vi "Convert Font To Font Object.vi"(8 "error in (no error)":errorcluster, 10 "Font":T1={"Name"="Calibri", "Size"=12, "Bold"=FALSE, "Italic"=FALSE, "Underline"=18, "Strike"=FALSE, "Color"=0} {"Underline" items=["Single"=1, "Words"=2, "Double"=3, "Thick"=4, "Dotted"=5, "DottedHeavy"=6, "Dash"=7, "DashedHeavy"=8, "DashLong"=9, "DashLongHeavy"=10, "DotDash"=11, "DashDotHeavy"=12, "DotDotDash"=13, "DashDotDotHeavy"=14, "Wave"=15, "WavyHeavy"=16, "WavyDouble"=17, "None"=18]}) -> (0 "error out":errorcluster, 3 "Font Object":refnum<class "Style.lvclass">)   [LabVIEW 2020, in "Styles.lvlib"]
uses:
  Styles.lvlib
  Style/Style.lvclass
  Title/Title.lvclass
  Heading 1/Heading 1.lvclass
  Heading 2/Heading 2.lvclass
  Heading 3/Heading 3.lvclass
  D:/Benjamin/Documents/Perso/Code/WC/LabVIEW_NPOI/src/Font/Font/Style.lvclass
  D:/Benjamin/Documents/Perso/Code/WC/LabVIEW_NPOI/src/Font/Title/Title.lvclass
  D:/Benjamin/Documents/Perso/Code/WC/LabVIEW_NPOI/src/Font/Heading/Heading.lvclass
  D:/Benjamin/Documents/Perso/Code/WC/LabVIEW_NPOI/src/Font/Heading 1/Heading 1.lvclass
  D:/Benjamin/Documents/Perso/Code/WC/LabVIEW_NPOI/src/Font/Heading 2/Heading 2.lvclass
  D:/Benjamin/Documents/Perso/Code/WC/LabVIEW_NPOI/src/Font/Heading 3/Heading 3.lvclass
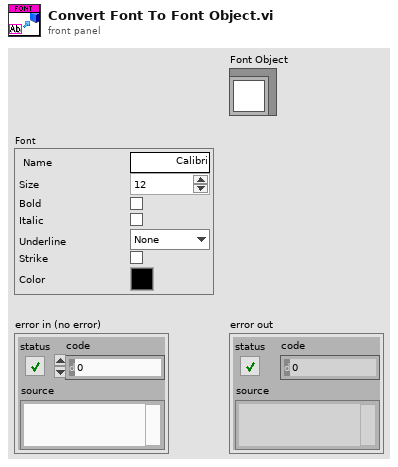
[diagram p1: front panel]
types:
  T1 = cluster{"Name":string, "Size":i32, "Bold":bool, "Italic":bool, "Underline":i32, "Strike":bool, "Color":u32}
  T2 = typedef "Styles.lvlib/Style.lvclass/Underline--ring.ctl" = i32
  T3 = cluster{"Public VIs:Properties:Name":string, "Public VIs:Properties:Size":i32, "Public VIs:Properties:Bold":bool, "Public VIs:Properties:Italic":bool, "Public VIs:Properties:Underline":T2, "Public VIs:Properties:Strike":bool, "Public VIs:Properties:Color":u32}
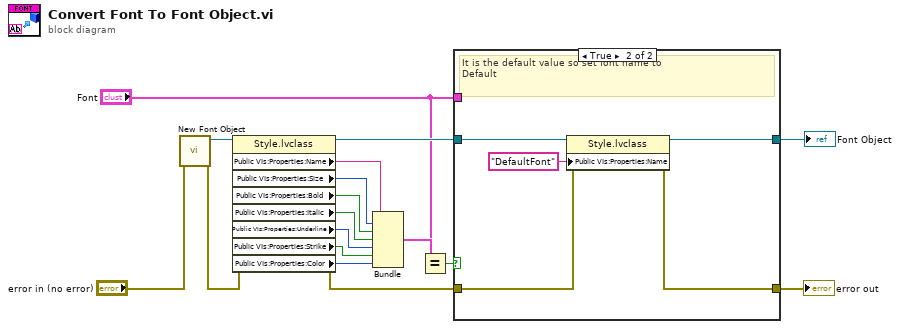
[diagram p0: block diagram]
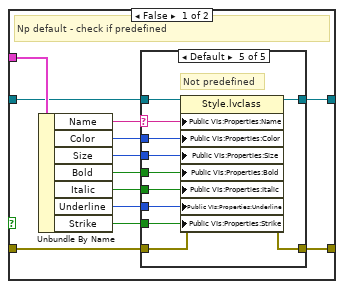
[diagram p2: hidden frame]
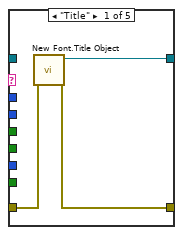
[diagram p3: hidden frame]
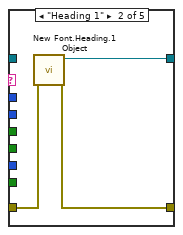
[diagram p4: hidden frame]
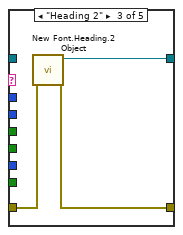
[diagram p5: hidden frame]
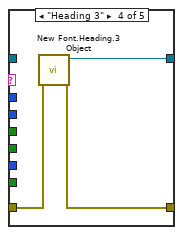
[diagram p6: hidden frame]
diagram:
  n1 = call "New Font Object.vi"("error in (no error)"="error in (no error)") -> ("error out"=w2:errorcluster, "Font out"=w4:refnum<class "Style.lvclass">)  [unwired: 9 in]
  n2 = property class="Style.lvclass"(reference=w4, error in=w2) -> (reference out=w14:refnum<class "Style.lvclass">, error out=w5:errorcluster, "Public VIs:Properties:Name"=w13:string, "Public VIs:Properties:Size"=w12:i32, "Public VIs:Properties:Bold"=w11:bool, "Public VIs:Properties:Italic"=w10:bool, "Public VIs:Properties:Underline"=w9:T2, "Public VIs:Properties:Strike"=w8:bool, "Public VIs:Properties:Color"=w7:u32)
  n3 = Bundle("Public VIs:Properties:Name"=w13, "Public VIs:Properties:Size"=w12, "Public VIs:Properties:Bold"=w11, "Public VIs:Properties:Italic"=w10, "Public VIs:Properties:Underline"=w9, "Public VIs:Properties:Strike"=w8, "Public VIs:Properties:Color"=w7) -> (w6:T3)  [unwired: 1 in]
  n4 = Equal?(x=w6, y="Font") -> (x = y?=w17:bool)
  n5 = case shown="True" w17 {
    tunnel: "Font" -> [w23 _]
    tunnel: [w22 w56] -> w16
    tunnel: w14 -> [w19 w57]
    tunnel: [w21 w54] -> w15
    tunnel: w5 -> [w18 w53]
    frame False {
      # "Np default - check if predefined"
      n6 = Unbundle By Name(w23) -> ("Name"=w20:string, "Color"=w28:u32, "Size"=w27:i32, "Bold"=w26:bool, "Italic"=w25:bool, "Underline"=w24:i32, "Strike"=w29:bool)
      n7 = case shown="Default" w20 {
        selector: w20 -> [_ _ _ _ w44]
        tunnel: w29 -> [_ _ _ _ w52]
        tunnel: w28 -> [_ _ _ _ w51]
        tunnel: w27 -> [_ _ _ _ w50]
        tunnel: w26 -> [_ _ _ _ w49]
        tunnel: w25 -> [_ _ _ _ w48]
        tunnel: w24 -> [_ _ _ _ w47]
        tunnel: [w32 w35 w38 w41 w46] -> w22
        tunnel: [w30 w33 w37 w39 w45] -> w21
        tunnel: w19 -> [_ _ _ _ w43]
        tunnel: w18 -> [w31 w34 w36 w40 w42]
        frame "Title" {
          n8 = call "New Font.Title Object.vi"("error in (no error)"=w31) -> ("error out"=w30:errorcluster, "Title out"=w32:refnum<class "Title.lvclass">)  [unwired: 9 in]
        }
        frame "Heading 1" {
          n9 = call "New Font.Heading.1 Object.vi"("error in (no error)"=w34) -> ("error out"=w33:errorcluster, "Heading 1 out"=w35:refnum<class "Heading 1.lvclass">)  [unwired: 9 in]
        }
        frame "Heading 2" {
          n10 = call "New Font.Heading.2 Object.vi"("error in (no error)"=w36) -> ("error out"=w37:errorcluster, "Heading 2 out"=w38:refnum<class "Heading 2.lvclass">)  [unwired: 9 in]
        }
        frame "Heading 3" {
          n11 = call "New Font.Heading.3 Object.vi"("error in (no error)"=w40) -> ("error out"=w39:errorcluster, "Heading 3 out"=w41:refnum<class "Heading 3.lvclass">)  [unwired: 9 in]
        }
        frame Default {
          # "Not predefined"
          # "Not predefined"
          n12 = property class="Style.lvclass"(reference=w43, error in=w42, "Public VIs:Properties:Name"=w44, "Public VIs:Properties:Color"=w51, "Public VIs:Properties:Size"=w50, "Public VIs:Properties:Bold"=w49, "Public VIs:Properties:Italic"=w48, "Public VIs:Properties:Underline"=w47, "Public VIs:Properties:Strike"=w52) -> (reference out=w46:refnum<class "Style.lvclass">, error out=w45:errorcluster)
        }
      }
    }
    frame True {
      # "It is the default value so set font name to \nDefault"
      n13 = property class="Style.lvclass"(reference=w57, error in=w53, "Public VIs:Properties:Name"="DefaultFont" ("Style:Name")) -> (reference out=w56:refnum<class "Style.lvclass">, error out=w54:errorcluster)
    }
  }
  "Font Object" <- w16
  "error out" <- w15
